vi "ConvertSCPIValueToBoolean.vi"(11 "SCPI Value":string) -> (3 "Boolean":bool)   [LabVIEW 2014, in "Keithley-6482-Visa.lvlib"]
uses:
  Keithley-6482-Visa.lvlib
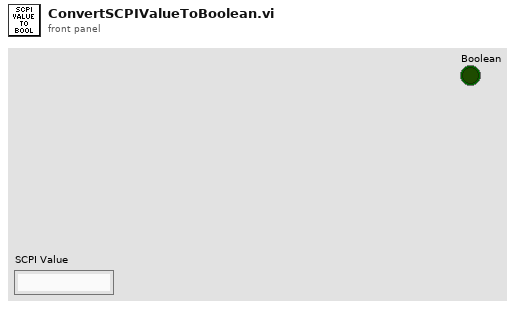
[diagram p1: front panel]
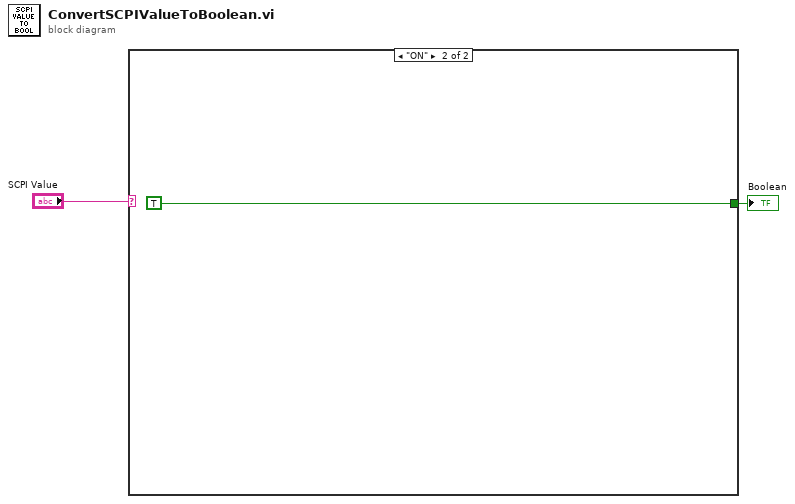
[diagram p0: block diagram]
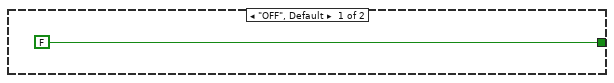
[diagram p2: hidden frame]
diagram:
  n1 = case shown="\"ON\"" "SCPI Value" {
    tunnel: [FALSE TRUE] -> w1
    frame "OFF", Default {
    }
    frame "ON" {
    }
  }
  "Boolean" <- w1
